vi "Calculate piezo V array.vi"(7 "N steps":i32=4, 8 "error in (no error)":errorcluster, 9 "Calib type":T1, 10 "2 PI":T2={"2 Pi Red"=1.65582, "2 Pi Green"=1.57699, "2 Pi Blue"=1.57699}, 11 "Initial voltage":sgl=0.7) -> (0 "error out":errorcluster, 3 "V array":sgl[][](array[numeric]))   [LabVIEW 2020]
uses:
  Controls/Calibration color ---typedef.ctl
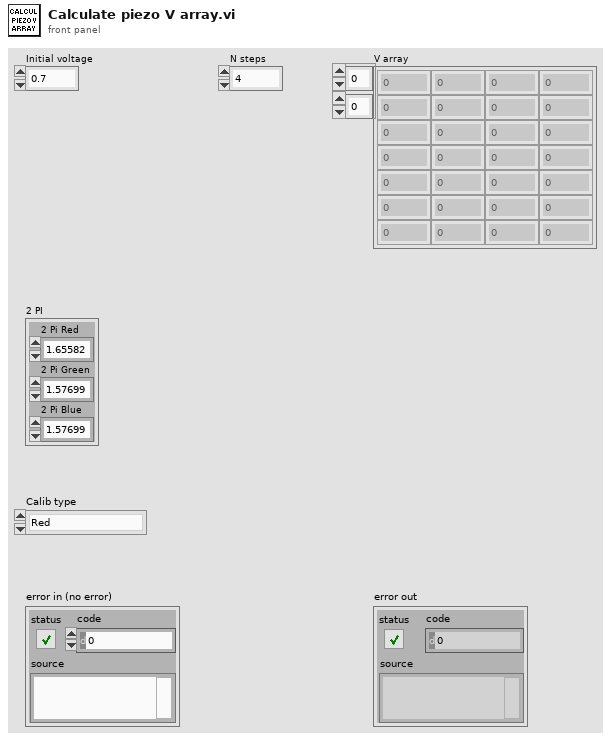
[diagram p1: front panel]
types:
  T1 = typedef "Calibration color ---typedef.ctl" = enum16{"Red", "Green", "Blue", "White", "All", "Reset", "Get"}
  T2 = cluster{"2 Pi Red":sgl, "2 Pi Green":sgl, "2 Pi Blue":sgl}
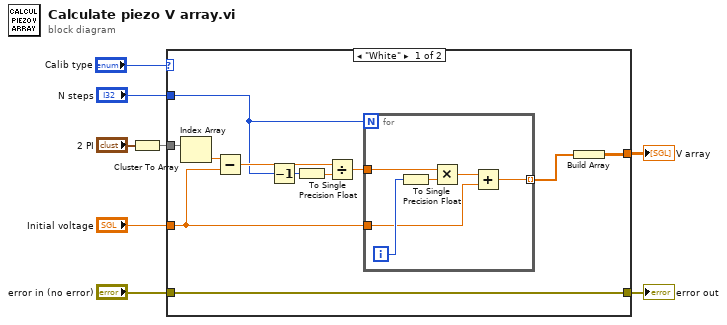
[diagram p0: block diagram]
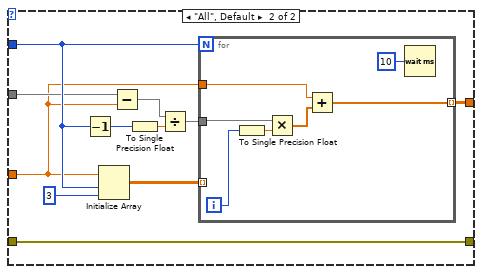
[diagram p2: hidden frame]
diagram:
  n1 = Cluster To Array(cluster="2 PI") -> (array=w5:sgl[])
  n2 = case shown="\"White\"" "Calib type" {
    tunnel: "N steps" -> [w14 w32]
    tunnel: [w9 w31] -> w6
    tunnel: w5 -> [w18 w29]
    tunnel: "Initial voltage" -> [w16 w27]
    tunnel: "error in (no error)" -> [w19 w26]
    tunnel: [w19 w26] -> w1
    frame "White" {
      n3 = Index Array(array=w18) -> (element=w17:sgl)  [unwired: 1 in]
      n4 = Subtract(x=w17, y=w16) -> (x-y=w15:sgl)
      n5 = Decrement(x=w14) -> (x-1=w12:i32)
      n6 = To Single Precision Float(number=w12) -> (single precision float=w13:sgl)
      n7 = Divide(x=w15, y=w13) -> (x/y=w11:sgl)
      n8 = for {
        N: w14 -> [_]
        tunnel: w16 -> [w21]
        tunnel: w11 -> [w25]
        tunnel: [w20] -> w10 mode=indexing
        i -> [w24]
        n9 = To Single Precision Float(number=w24) -> (single precision float=w23:sgl)
        n10 = Multiply(x=w25, y=w23) -> (x*y=w22:sgl)
        n11 = Add(x=w22, y=w21) -> (x+y=w20:sgl)
      }
      n12 = Build Array(w10) -> (w9:sgl[][])
    }
    frame "All", Default {
      n13 = Decrement(x=w32) -> (x-1=w30:i32)
      n14 = Initialize Array(w27, w32, 3 ("dimension size")) -> (w36:sgl[][])
      n15 = Subtract(x=w29, y=w27) -> (x-y=w28:sgl[])
      n16 = To Single Precision Float(number=w30) -> (single precision float=w35:sgl)
      n17 = Divide(x=w28, y=w35) -> (x/y=w34:sgl[])
      n18 = for {
        N: w32 -> [_]
        tunnel: w36 -> [_] mode=indexing
        tunnel: w34 -> [w41]
        tunnel: w27 -> [w42]
        tunnel: [w37] -> w31 mode=indexing
        i -> [w40]
        n19 = To Single Precision Float(number=w40) -> (single precision float=w38:sgl)
        n20 = Multiply(x=w41, y=w38) -> (x*y=w39:sgl[])
        n21 = Add(x=w42, y=w39) -> (x+y=w37:sgl[])
        n22 = Wait (ms)(milliseconds to wait=u32 10) -> ()  [unwired: 1 out]
      }
    }
  }
  "V array" <- w6
  "error out" <- w1
